vi "Global.vi"() -> ()   [LabVIEW 2019]
panel:
  out "Sensor signal":dbl
  in  "Actuator Signal - R":bool
  in  "Actuator Signal - L":bool
  out "Bending Angle":cluster{"L&R":dbl, "Envelope":dbl}
  out "Sensor Angles":cluster{"Left":dbl, "Right":dbl}
  out "Solenoid":cluster{"Solenoid 1":bool, "Solenoid 2":bool}
  out "Ref":dbl
  out "Angle rad":dbl
  out "Angle 2":dbl
  in  "off/on":bool
  out "outy":dbl
  out "Sensor Raw Voltage":cluster{"Left":dbl, "Right":dbl}
  out "Sensors":cluster{"Sensor 1":dbl, "Sensor 2":dbl}
  in  "Regulator off/on":bool
  out "Sin wave element":dbl
  in  "Sin wave":T1={"Frequency (Hz)"=0.0, "Amplitude"=0.0, "Phase"=5.0}
  out "Angle":dbl
  in  "Square wave":T2
  out "regulator on/off":bool
  in  "Stop Button":bool
  in  "Actuator freq":dbl
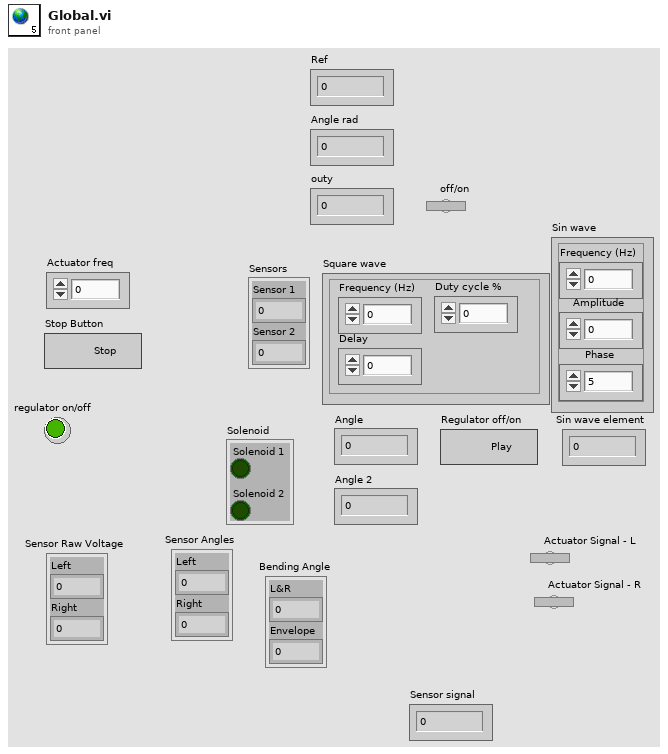
[diagram p1: front panel]
types:
  T1 = cluster{"Frequency (Hz)":dbl, "Amplitude":dbl, "Phase":dbl}
  T2 = cluster{"Frequency (Hz)":dbl, "Delay":dbl, "Duty cycle %":dbl}
diagram:
